vi "GetLimits.vi"(8 "entrée d'erreur (pas d'erreur)":errorcluster, 10 "Axis":T1 items=["1"=1, "2"=2, "3"=3, "4"=4], 11 "DelayLineLS4 en entrée":refnum<class "DelayLineLS4.lvclass">) -> (0 "error out":errorcluster, 1 "max":dbl, 2 "min":dbl, 3 "DelayLineLS4 out":refnum<class "DelayLineLS4.lvclass">)   [LabVIEW 2015, in "DelayLineLS4.lvclass"]
uses:
  DelayLineLS4.lvclass
  LS4 axis.ctl
  LS4_parameters.ctl
  GeneralFunctionality/GeneralFunctionality.lvclass/GeneralFunctionality.ctl
  Config/Config.lvclass
  DelayLine.lvclass
  GeneralFunctionality/GeneralFunctionality.lvclass
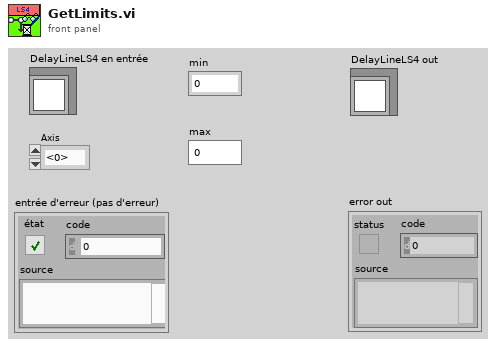
[diagram p1: front panel]
types:
  T1 = typedef "DelayLine.lvclass/LS4 axis.ctl" = u16
  T2 = typedef "DelayLine.lvclass/LS4_parameters.ctl" = string
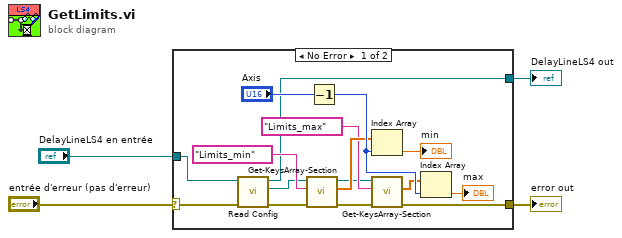
[diagram p0: block diagram]
diagram:
  n1 = case shown="No Error" "entrée d'erreur (pas d'erreur)" {
    selector: "entrée d'erreur (pas d'erreur)" -> [w5 w22]
    tunnel: "DelayLineLS4 en entrée" -> [w8 w21]
    tunnel: [w7 w21] -> w3
    tunnel: [w6 w22] -> w2
    frame No Error {
      n2 = call "Read Config.vi"("error in (no error)"=w5, "GeneralFunctionality en entrée"=w8) -> ("error out"=w10:errorcluster, "Config.lvclass"=w9:refnum<class "Config.lvclass">, "GeneralFunctionality en sortie"=w7:refnum<class "DelayLineLS4.lvclass">)  [unwired: 7 in]
      n3 = call "Get-KeysArray-Section.vi"("error in (no error)"=w10, "Section"=T2 "Limits_min", "Config in"=w9) -> ("error out"=w13:errorcluster, "Array"=w16:dbl[], "Config out"=w12:refnum<class "Config.lvclass">)  [unwired: 6 in]
      n4 = Decrement(x="Axis") -> (x-1=w18:T1)
      n5 = Index Array(array=w16, index=w18) -> (element=→"min":dbl)
      n6 = call "Get-KeysArray-Section.vi"("error in (no error)"=w13, "Section"=T2 "Limits_max", "Config in"=w12) -> ("error out"=w6:errorcluster, "Array"=w15:dbl[])  [unwired: 6 in, 1 out]
      n7 = Index Array(array=w15, index=w18) -> (element=→"max":dbl)
    }
    frame Error {
    }
  }
  "DelayLineLS4 out" <- w3
  "error out" <- w2
